vi "Acquire Data - Config.vi"(7 "Total Buffer Size":i32, 8 "error in (no error)":errorcluster, 10 "Acquisition Data v1":T1={"Data Rate"=1, "Samples per Read"=0, "Number of Reads to Save"=0, "Data File Name"="", "TDMS Properties"=[], "Number of Channels"=4, "Channel Scale Array"=[0.0, 0.0, 0.0, 0.0, 0.0, 0.0, 0.0, 0.0, 0.0, 0.0, 0.0, 0.0, 0.0, 0.0, 0.0, 0.0, 0.0, 0.0, 0.0, 0.0, 0.0, 0.0, 0.0, 0.0], "Channel Names"=[], "Trigger - RMS Value"=0.0, "Trigger - Channel"=0, "Trigger - Time (Minute)"=0, "Input Configuration"=0} {"Input Configuration" items=["AC Coupled", "DC Coupled", "IEPE AC Coupled"]; "Data Rate" items=["51.200 kS/s (NI 9234)"=1, "25.600 kS/s (NI 9234)"=2, "17.067 kS/s (NI 9234)"=3, "12.800 kS/s (NI 9234)"=4, "10.240 kS/s (NI 9234)"=5, "8.533 kS/s (NI 9234)"=6, "7.314 kS/s (NI 9234)"=7, "6.400 kS/s (NI 9234)"=8, "5.689 kS/s (NI 9234)"=9, "5.120 kS/s (NI 9234)"=10, "4.654 kS/s (NI 9234)"=11, "4.267 kS/s (NI 9234)"=12, "3.938 kS/s (NI 9234)"=13, "3.657 kS/s (NI 9234)"=14, "3.413 kS/s (NI 9234)"=15, "3.200 kS/s (NI 9234)"=16, "3.012 kS/s (NI 9234)"=17, "2.845 kS/s (NI 9234)"=18, "2.695 kS/s (NI 9234)"=19, "2.560 kS/s (NI 9234)"=20, "2.438 kS/s (NI 9234)"=21, "2.328 kS/s (NI 9234)"=22, "2.226 kS/s (NI 9234)"=23, "2.133 kS/s (NI 9234)"=24, "2.048 kS/s (NI 9234)"=25, "1.969 kS/s (NI 9234)"=26, "1.896 kS/s (NI 9234)"=27, "1.829 kS/s (NI 9234)"=28, "1.765 kS/s (NI 9234)"=29, "1.707 kS/s (NI 9234)"=30, "1.652 kS/s (NI 9234)"=31]}, 11 "FPGA VI Reference":T5) -> (0 "error out":errorcluster, 1 "Waveform Data":waveform(sgl)[](array[waveform]))   [LabVIEW 2015]
doc: "Reads waveform data from the DMA FIFO."
uses:
  controls/FPGA VI Reference.ctl
  controls/Acquisition and Logging Configuration_v1.ctl
  <vilib>/LabVIEW Targets/FPGA/cRIO/shared/nicrio_ModuleControls/nicrio_cRIO-9234_DataRatesRing2.ctl
  controls/TDMS Properties.ctl
  <vilib>/LabVIEW Targets/FPGA/cRIO/shared/nicrio_ModuleControls/nicrio_cRIO-9234_ConfigModeRing.ctl
  <vilib>/Utility/error.llb/Error Cluster From Error Code.vi
  <vilib>/rvi/errors/niLvFpgaAdjustHostInterfaceError.vi
  Globals/Global - Monitoring Variables.vi
  <vilib>/rvi/interface/nirviReadWriteControl/nirviReadWriteControl.xnode
  <vilib>/rvi/interface/nirviMethod/nirviMethod.xnode
  NiFpgaLv.dll
  <vilib>/rvi/interface/Simulation/niFpgaSimulationCallBeginRW.vi
  <vilib>/FPGAPlugInAG/Dynamic/niLvFpga_ReadFifo_Dynamic.vi
  <vilib>/rvi/errors/niLvFpgaMergeErrorWithErrorCode.vi
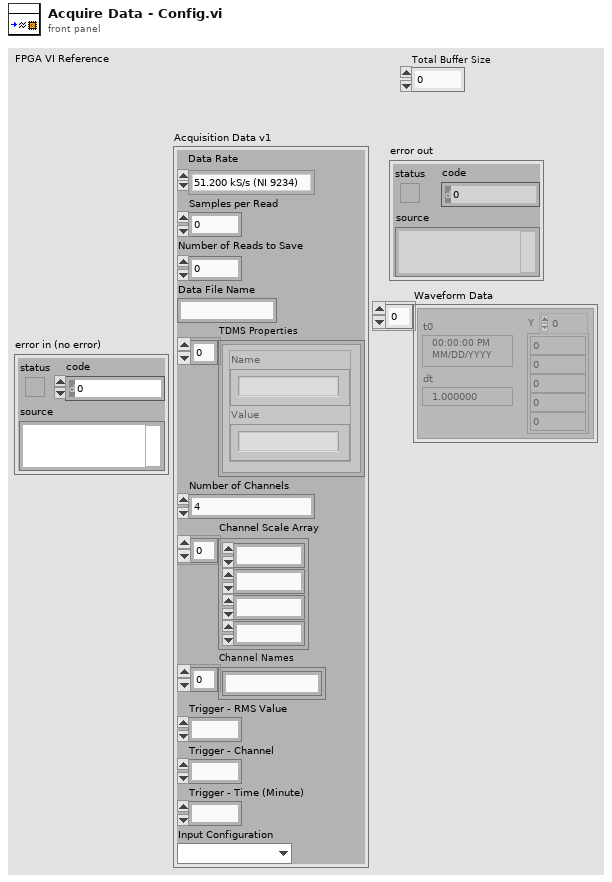
[diagram p1: front panel]
types:
  T1 = typedef "Acquisition and Logging Configuration_v1.ctl" = cluster{"Data Rate":T2, "Samples per Read":i32, "Number of Reads to Save":i32, "Data File Name":string, "TDMS Properties":T3[], "Number of Channels":i32, "Channel Scale Array":fxp<+,24,12>[], "Channel Names":string[], "Trigger - RMS Value":dbl, "Trigger - Channel":i32, "Trigger - Time (Minute)":i32, "Input Configuration":T4}
  T2 = typedef "nicrio_cRIO-9234_DataRatesRing2.ctl" = u8
  T3 = typedef "TDMS Properties.ctl" = cluster{"Name":string, "Value":string}
  T4 = typedef "nicrio_cRIO-9234_ConfigModeRing.ctl" = u8
  T5 = typedef "FPGA VI Reference.ctl" = refnum<k20>
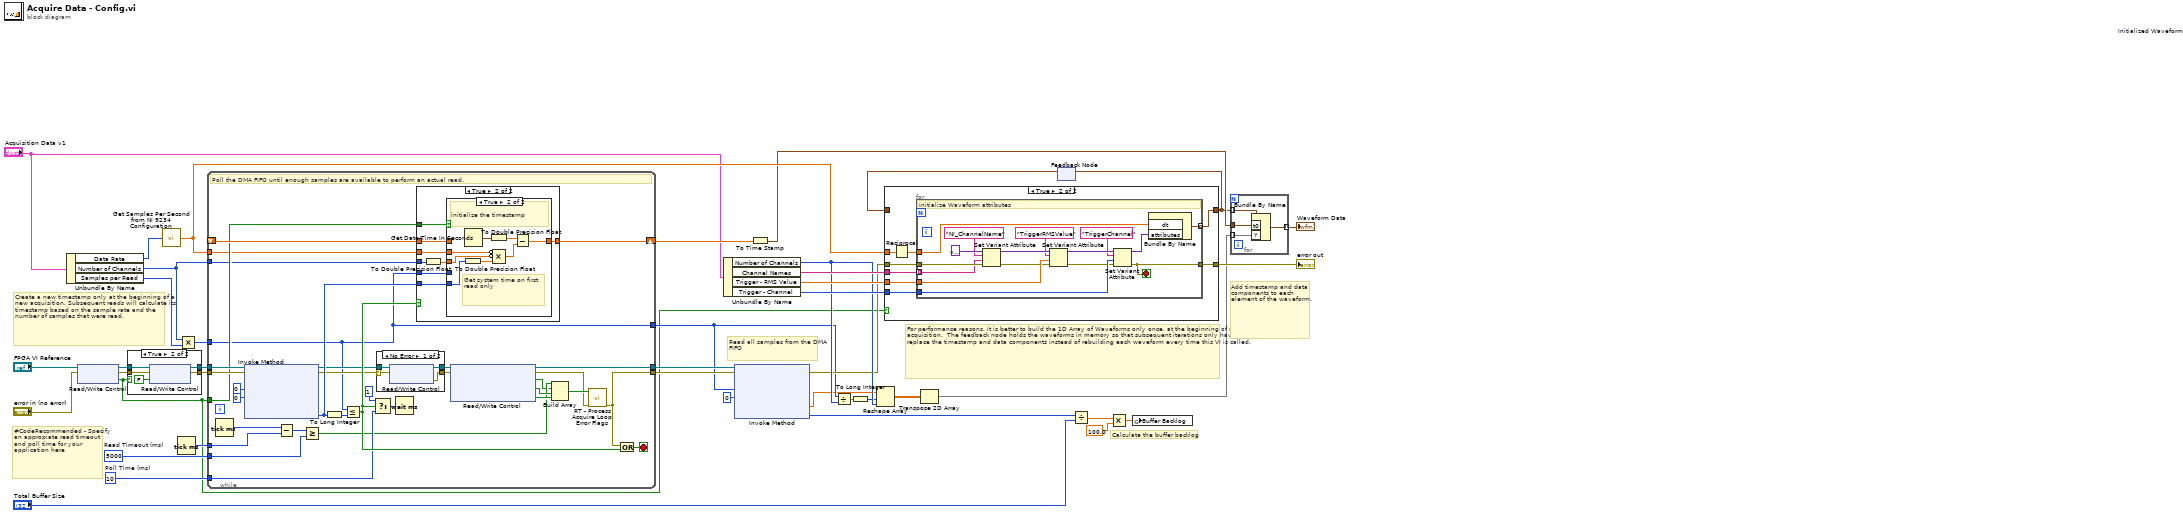
[diagram p0: block diagram]
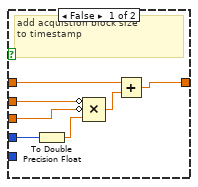
[diagram p5: hidden frame]
diagram:
  w17 = u32 10  # Poll Time (ms)
  w18 = u32 5000  # Read Timeout (ms)
  # "Calculate the buffer backlog"
  # "For performance reasons, it is better to build the 1D Array of Waveforms only once, at the beginning of an acquisition.  The feedback node holds the waveforms in memory so that subsequent iterations only have to replace the timestamp and data components instead of rebuilding each waveform every time this VI is called."
  # "Read all samples from the DMA FIFO"
  # "#CodeRecommended - Specify an appropiate read timeout and poll time for your application here"
  # "Create a new timestamp only at the beginning of a new acquisition. Subsequent reads will calculate its timestamp based on the sample rate and the number of samples that were read."
  # "Add timestamp and data components to each element of the waveform."
  n1 = Unbundle By Name("Acquisition Data v1") -> ("Data Rate"=w5:T2, "Number of Channels"=w3:i32, "Samples per Read"=w4:i32)
  n2 = xnode "Read/Write Control"("FPGA VI Reference In"="FPGA VI Reference", "error in"="error in (no error)") -> ("FPGA VI Reference Out"=w39:T5, "error out"=w40:errorcluster, "First Read"=w12:bool)
  n3 = case shown="True" w12 {
    tunnel: w39 -> [w43 w48]
    tunnel: [w43 w47] -> w37
    tunnel: w40 -> [w42 w46]
    tunnel: [w42 w45] -> w36
    frame False {
    }
    frame True {
      n4 = xnode "Read/Write Control"("FPGA VI Reference In"=w48, "error in"=w46, "First Read"=FALSE) -> ("FPGA VI Reference Out"=w47:T5, "error out"=w45:errorcluster)
    }
  }
  n5 = call "Get Samples Per Second from NI 9234 Configuration.vi"("Sample Rate (51.2k )"=w5) -> ("Samples per second"=w41:dbl)  [unwired: 4 in]
  n6 = Tick Count (ms)() -> (millisecond timer value=w35:u32)
  n7 = Multiply(x=w3, y=w4) -> (x*y=w27:i32)
  n8 = while {
    tunnel: [w53] -> w33
    tunnel: [w59] -> w34
    tunnel: w12 -> [w76]
    tunnel: w37 -> [w79]
    tunnel: w36 -> [w78]
    shift-right: [w71] -> w31
    shift-left: _ -> [w77]
    tunnel: w35 -> [w80]
    tunnel: w27 -> [w49]
    tunnel: [w49] -> w16
    tunnel: w3 -> [w50]
    tunnel: w18 -> [w65]
    tunnel: w17 -> [w64]
    tunnel: w41 -> [w51]
    stop <- w81 stop-if-true
    # "Poll the DMA FIFO until enough samples are available to perform an actual read."
    n9 = Tick Count (ms)() -> (millisecond timer value=w75:u32)
    n10 = xnode "Invoke Method"("FPGA VI Reference In"=w79, "error in"=w78, "Number of Elements"=u32 0, "Timeout (ms)"=0) -> ("FPGA VI Reference Out"=w62:T5, "error out"=w63:errorcluster, "Elements Remaining"=w67:u32)  [unwired: 1 out]
    n11 = Subtract(x=w75, y=w80) -> (x-y=w66:u32)
    n12 = Greater Or Equal?(x=w66, y=w65) -> (x >= y?=w56:bool)
    n13 = To Long Integer(number=w67) -> (32bit integer=w70:i32)
    n14 = Less Or Equal?(x=w49, y=w70) -> (x <= y?=w74:bool)
    n15 = Select(t=u32 1, s=w74, f=w64) -> (s? t:f=w73:u32)
    n16 = case shown="No Error" w63 {
      selector: w63 -> [w85 w86]
      tunnel: w62 -> [w84 w87]
      tunnel: [w83 w87] -> w61
      tunnel: [w82 w86] -> w60
      frame No Error {
        n17 = xnode "Read/Write Control"("FPGA VI Reference In"=w84, "error in"=w85) -> ("FPGA VI Reference Out"=w83:T5, "FPGA Error"=w82:errorcluster)  [unwired: 1 out]
      }
      frame Error {
      }
    }
    n18 = Wait (ms)(milliseconds to wait=w73) -> ()  [unwired: 1 out]
    n19 = case shown="True" w74 {
      tunnel: w77 -> [w88 w96]
      tunnel: w76 -> [_ w95]
      tunnel: w67 -> [_ w94]
      tunnel: [w88 w93] -> w71
      tunnel: w49 -> [_ w92]
      tunnel: w51 -> [_ w90]
      tunnel: w50 -> [_ w89]
      frame False {
      }
      frame True {
        n20 = To Double Precision Float(number=w89) -> (double precision float=w91:dbl)
        n21 = case shown="True" w95 {
          tunnel: w90 -> [w101 w111]
          tunnel: w96 -> [w102 _]
          tunnel: w92 -> [w98 _]
          tunnel: w91 -> [w99 w110]
          tunnel: w94 -> [_ w105]
          tunnel: [w103 w107] -> w93
          frame False {
            # "add acquistion block size\nto timestamp"
            n22 = To Double Precision Float(number=w98) -> (double precision float=w97:dbl)
            n23 = Compound Arithmetic op=MULTIPLY(invert w101, invert w99, w97) -> (w100:dbl)
            n24 = Add(x=w102, y=w100) -> (x+y=w103:dbl)
          }
          frame True {
            # "Get system time on first read only"
            # "initialize the timestamp"
            n25 = To Double Precision Float(number=w105) -> (double precision float=w104:dbl)
            n26 = Get Date/Time In Seconds() -> (seconds since 1Jan1904=w109:timestamp)
            n27 = To Double Precision Float(number=w109) -> (double precision float=w106:dbl)
            n28 = Compound Arithmetic op=MULTIPLY(invert w111, invert w110, w104) -> (w108:dbl)
            n29 = Subtract(x=w106, y=w108) -> (x-y=w107:dbl)
          }
        }
      }
    }
    n30 = xnode "Read/Write Control"("FPGA VI Reference In"=w61, "error in"=w60) -> ("FPGA VI Reference Out"=w59:T5, "error out"=w52:errorcluster, "Module Underflow"=w55:bool, "DMA FIFO Full"=w58:bool, "Different Channel Count"=w57:bool)
    n31 = Build Array(w56, w55, w58, w57) -> (w54:bool[])
    n32 = call "RT - Process Acquire Loop Error Flags.vi"("error in (no error)"=w52, "Error Flags"=w54) -> ("error out"=w53:errorcluster)  [unwired: 9 in]
    n33 = Compound Arithmetic op=OR(w53, w74) -> (w81:bool)
  }
  n34 = Unbundle By Name("Acquisition Data v1") -> ("Number of Channels"=w26:i32, "Channel Names"=w28:string[], "Trigger - RMS Value"=w29:dbl, "Trigger - Channel"=w32:i32)
  n35 = xnode "Invoke Method"("FPGA VI Reference In"=w34, "error in"=w33, "Number of Elements"=w16, "Timeout (ms)"=0) -> ("error out"=w20:errorcluster, "Data"=w6:sgl[], "Elements Remaining"=w10:u32)  [unwired: 1 out]
  n36 = To Time Stamp(1:w31) -> (0:w15:timestamp)
  n37 = Divide(x=w16, y=w26) -> (x/y=w25:dbl)
  n38 = To Long Integer(number=w25) -> (32bit integer=w24:i32)
  n39 = Reshape Array(w6, w24, w26) -> (w23:sgl[][])
  n40 = Transpose 2D Array(2D array=w23) -> (transposed array=w22:sgl[][])
  n41 = feedback #1 "Initialized Waveforms"() -> (w13:waveform(sgl)[])  [unwired: 1 in]
  n42 = case shown="True" w12 {
    tunnel: w32 -> [_ w121]
    tunnel: w20 -> [w113 w120]
    tunnel: [w113 w119] -> w30
    tunnel: w29 -> [_ w118]
    tunnel: w28 -> [_ w117]
    tunnel: [w112 w116] -> w14
    tunnel: w13 -> [w112 _]
    tunnel: w41 -> [_ w115]
    frame False {
    }
    frame True {
      n43 = Reciprocal(x=w115) -> (1/x=w114:dbl)
      n44 = for {
        tunnel: w114 -> [w137]
        tunnel: [w136] -> w116 mode=indexing
        tunnel: w118 -> [w134]
        tunnel: w121 -> [w132]
        tunnel: w120 -> [w133]
        tunnel: [w122] -> w119
        tunnel: w117 -> [w123] mode=indexing
        stop <- w122 stop-if-true
        # "Initialize Waveform attributes"
        n45 = Set Variant Attribute(Variant=variant ("variant out"), name="NI_ChannelName", value=w123, error in=w133) -> (Variant out=w128:variant, error out=w130:errorcluster)  [unwired: 1 out]
        n46 = Set Variant Attribute(Variant=w128, name="TriggerRMSValue", value=w134, error in=w130) -> (Variant out=w129:variant, error out=w131:errorcluster)  [unwired: 1 out]
        n47 = Set Variant Attribute(Variant=w129, name="TriggerChannel", value=w132, error in=w131) -> (Variant out=w135:variant, error out=w122:errorcluster)  [unwired: 1 out]
        n48 = Bundle By Name("dt"=w137, "attributes"=w135) -> (w136:waveform(sgl))  [unwired: 1 out]
      }
    }
  }
  "error out" <- w30
  n49 = feedback-in #1(w14) -> ()
  n50 = Divide(x=w10, y="Total Buffer Size") -> (x/y=w11:dbl)
  n51 = Multiply(x=w11, y=100.0) -> (x*y=w8:dbl)
  n52 = global write "Global - Monitoring Variables.vi" "Buffer Backlog"(w8) -> ()
  n53 = for {
    tunnel: w14 -> [w141] mode=indexing
    tunnel: w15 -> [w140]
    tunnel: [w139] -> w2 mode=indexing
    tunnel: w22 -> [w138] mode=indexing
    n54 = Bundle By Name(cluster=w141, "t0"=w140, "Y"=w138) -> (w139:waveform(sgl))
  }
  "Waveform Data" <- w2
